vi "Employee Info to Variant Array.vi"(8 "error in (no error)":errorcluster caption="错误输入（无错误）", 10 "Employee Info":T1, 11 "Employee 输入":refnum<class "Employee.lvclass"> caption="DNL_LabVIEW Object in") -> (0 "error out":errorcluster caption="错误输出", 2 "Employee Info Var Array":variant[](array[variant]), 3 "Employee 输出":refnum<class "Employee.lvclass"> caption="DNL_LabVIEW Object out")   [LabVIEW 2012, in "Employee.lvclass"]
uses:
  Employee.lvclass
  Custom Def/Employee Info.ctl
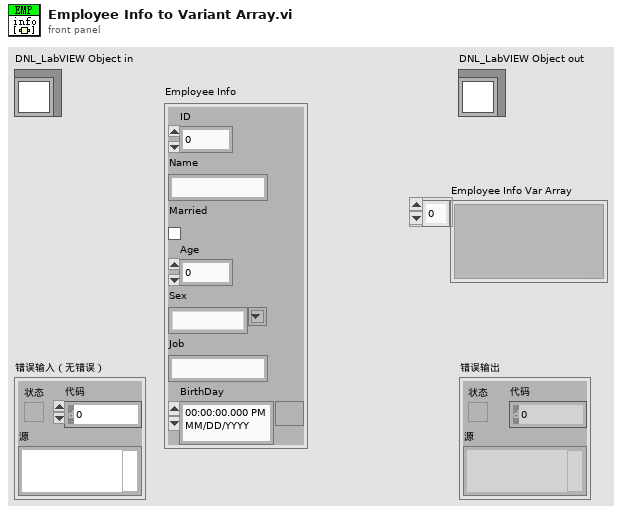
[diagram p1: front panel]
types:
  T1 = typedef "Employee Info.ctl" = cluster{"ID":u16, "Name":string, "Married":bool, "Age":u8, "Sex":string, "Job":string, "BirthDay":timestamp}
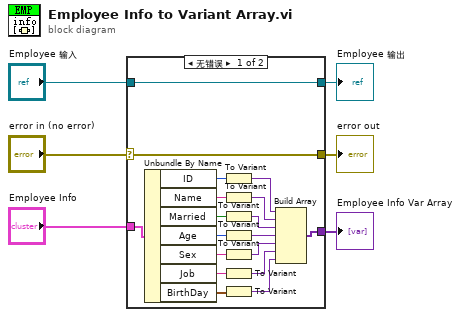
[diagram p0: block diagram]
diagram:
  n1 = case shown="无错误" "error in (no error)" {
    selector: "error in (no error)" -> [w23 w26]
    tunnel: [w23 w26] -> w5
    tunnel: [w24 w25] -> w3
    tunnel: "Employee 输入" -> [w24 w25]
    tunnel: "Employee Info" -> [w11 _]
    tunnel: [w10 _] -> w1
    frame No Error {
      n2 = Unbundle By Name(w11) -> ("ID"=w12:u16, "Name"=w13:string, "Married"=w14:bool, "Age"=w15:u8, "Sex"=w16:string, "Job"=w9:string, "BirthDay"=w8:timestamp)
      n3 = To Variant(anything=w12) -> (Variant=w17:variant)
      n4 = To Variant(anything=w13) -> (Variant=w18:variant)
      n5 = To Variant(anything=w14) -> (Variant=w19:variant)
      n6 = To Variant(anything=w15) -> (Variant=w20:variant)
      n7 = To Variant(anything=w16) -> (Variant=w21:variant)
      n8 = To Variant(anything=w9) -> (Variant=w22:variant)
      n9 = To Variant(anything=w8) -> (Variant=w7:variant)
      n10 = Build Array(w17, w18, w19, w20, w21, w22, w7) -> (w10:variant[])
    }
    frame Error {
    }
  }
  "error out" <- w5
  "Employee 输出" <- w3
  "Employee Info Var Array" <- w1
